vi "initialize.vi"(8 "error in (no error)":errorcluster, 9 "Default Goal Amount":dbl, 10 "Name":string, 11 "Category":refnum<class "Category.lvclass">) -> (0 "error out":errorcluster, 3 "Category out":refnum<class "Category.lvclass">)   [LabVIEW 2018, in "Category.lvclass"]
uses:
  Category.lvclass
  Category.lvclass/Category.ctl
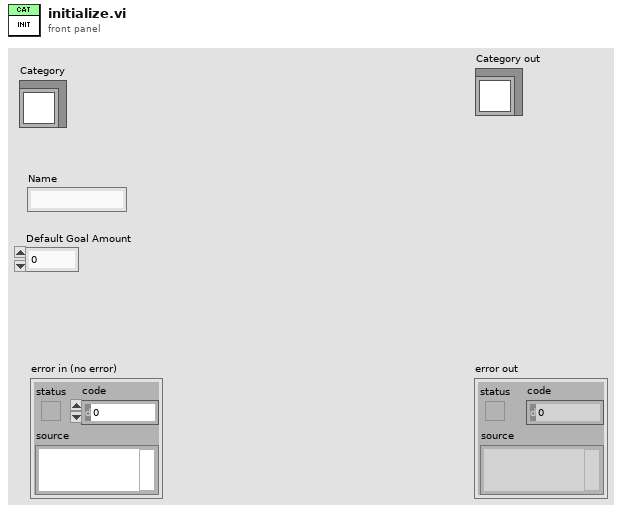
[diagram p1: front panel]
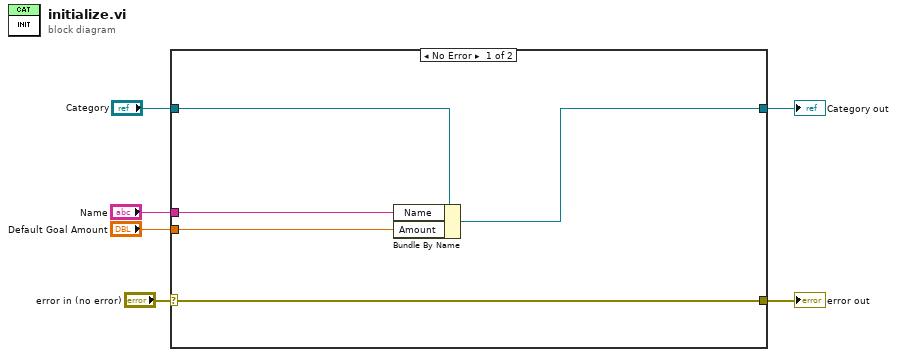
[diagram p0: block diagram]
diagram:
  n1 = case shown="No Error" "error in (no error)" {
    selector: "error in (no error)" -> [w9 w13]
    tunnel: [w9 w13] -> w5
    tunnel: [w10 w12] -> w4
    tunnel: "Category" -> [w11 w12]
    tunnel: "Default Goal Amount" -> [w8 _]
    tunnel: "Name" -> [w7 _]
    frame No Error {
      n2 = Bundle By Name(cluster=w11, "Name"=w7, "Amount"=w8) -> (w10:refnum<class "Category.lvclass">)
    }
    frame Error {
    }
  }
  "error out" <- w5
  "Category out" <- w4
